vi "Write Start index.vi"(8 "error in (no error)":errorcluster, 10 "Start index":i32, 11 "Acquis params in":refnum<class "CV-Acquisition.lvclass">) -> (0 "error out":errorcluster, 3 "Acquis params out":refnum<class "CV-Acquisition.lvclass">)   [LabVIEW 2013, in "CameraVision.lvlib" / "CV-Acquisition.lvclass"]
uses:
  CV-Acquisition.lvclass
  CV-Acquisition.lvclass/CV-Acquisition.ctl
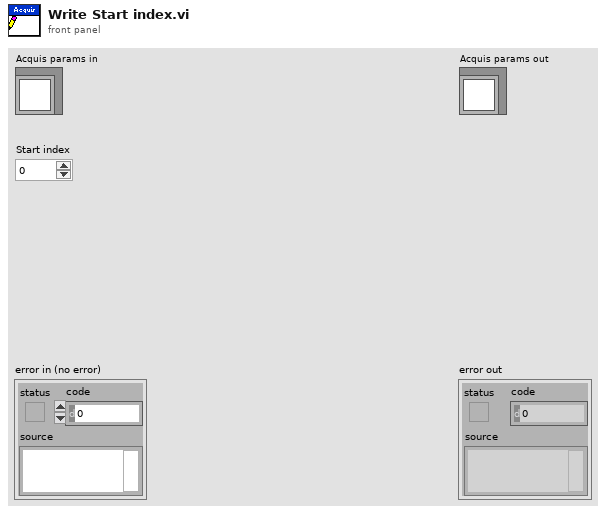
[diagram p1: front panel]
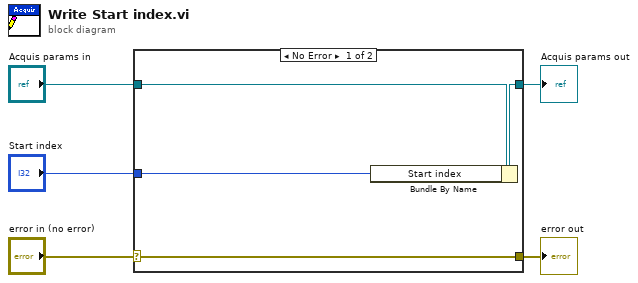
[diagram p0: block diagram]
diagram:
  n1 = case shown="No Error" "error in (no error)" {
    selector: "error in (no error)" -> [w9 w10]
    tunnel: [w9 w10] -> w4
    tunnel: [w7 w11] -> w2
    tunnel: "Acquis params in" -> [w8 w11]
    tunnel: "Start index" -> [w6 _]
    frame No Error {
      n2 = Bundle By Name(cluster=w8, "Start index"=w6) -> (w7:refnum<class "CV-Acquisition.lvclass">)
    }
    frame Error {
    }
  }
  "error out" <- w4
  "Acquis params out" <- w2
